vi "StoreEvents.vi"(8 "error in (no error)":errorcluster, 11 "PredictiveMaintenance.lvlib:PredictiveMaintenance_IN":refnum<class "PredictiveMaintenance.lvclass">) -> (0 "error out":errorcluster, 3 "PredictiveMaintenance.lvlib:PredictiveMaintenance_OUT":refnum<class "PredictiveMaintenance.lvclass">)   [LabVIEW 2019, in "PredictiveMaintenance.lvlib" / "PredictiveMaintenance.lvclass"]
uses:
  PredictiveMaintenance.lvclass
  PredictiveMaintenance.lvclass/PredictiveMaintenance.ctl
  ConfigClass/ConfigClass/ConfigClass.lvclass
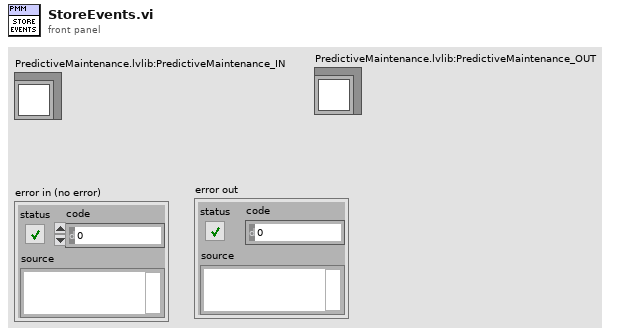
[diagram p1: front panel]
types:
  T1 = typedef "PredictiveMaintenance.lvlib/PredictiveMaintenance.lvclass/EventData.ctl" = cluster{"event":string, "curr_val":dbl, "warn_limit":dbl, "err_limit":dbl}
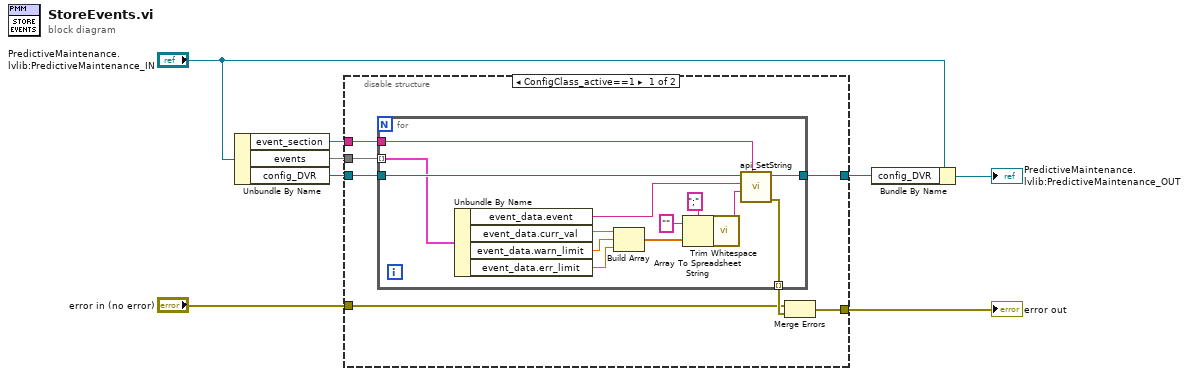
[diagram p0: block diagram]
diagram:
  n1 = Unbundle By Name("PredictiveMaintenance.lvlib:PredictiveMaintenance_IN") -> ("event_section"=w6:string, "events"=w8:map{string, T1}, "config_DVR"=w7:refnum<data-value>)
  n2 = disable-structure shown="ConfigClass_active==1" {
    disable-tunnel: w8 -> [w15 _]
    disable-tunnel: w7 -> [w14 w31]
    disable-tunnel: w6 -> [w13 _]
    disable-tunnel: [w11 w30] -> w5
    disable-tunnel: "error in (no error)" -> [w10 w30]
    disable-tunnel: [w9 w31] -> w2
    frame condition #0 (active) {
      n3 = for {
        tunnel: w15 -> [w27] mode=indexing
        tunnel: w14 -> [w29]
        tunnel: w13 -> [w28]
        tunnel: [w18] -> w12 mode=indexing
        tunnel: [w17] -> w9
        n4 = Unbundle By Name(w27) -> ("event_data.event"=w26:string, "event_data.curr_val"=w23:dbl, "event_data.warn_limit"=w22:dbl, "event_data.err_limit"=w21:dbl)
        n5 = Build Array(w23, w22, w21) -> (w20:dbl[])
        n6 = Array To Spreadsheet String(delimiter (Tab)=";", array=w20, 3:"" ("format string")) -> (spreadsheet string=w19:string)
        n7 = call <vilib>:"Trim Whitespace.vi"("string"=w19) -> ("trimmed string"=w16:string)  [unwired: 1 in]
        n8 = call "api_SetString.vi"("group"=w28, "string_in"=w16, "param"=w26, "ConfigClass_DVR"=w29) -> ("error out"=w18:errorcluster, "ConfigClass_DVR_out"=w17:refnum<data-value>)  [unwired: 6 in]
      }
      n9 = Merge Errors(w10, w12) -> (w11:errorcluster)
    }
    frame condition #1 {
    }
  }
  "error out" <- w5
  n10 = Bundle By Name(cluster="PredictiveMaintenance.lvlib:PredictiveMaintenance_IN", "config_DVR"=w2) -> (→"PredictiveMaintenance.lvlib:PredictiveMaintenance_OUT":refnum<class "PredictiveMaintenance.lvclass">)
